vi "Calulate Fluid Level.vi"(8 "error in (no error)":errorcluster, 11 "Model Data":T1) -> (0 "error out":errorcluster, 3 "Model Data Out":T1)   [LabVIEW 2016, in "Model.lvlib"]
uses:
  Model.lvlib
  TypeDefs/Model Data.ctl
  TypeDefs/PL Settings.ctl
  TypeDefs/PL UI Refs.ctl
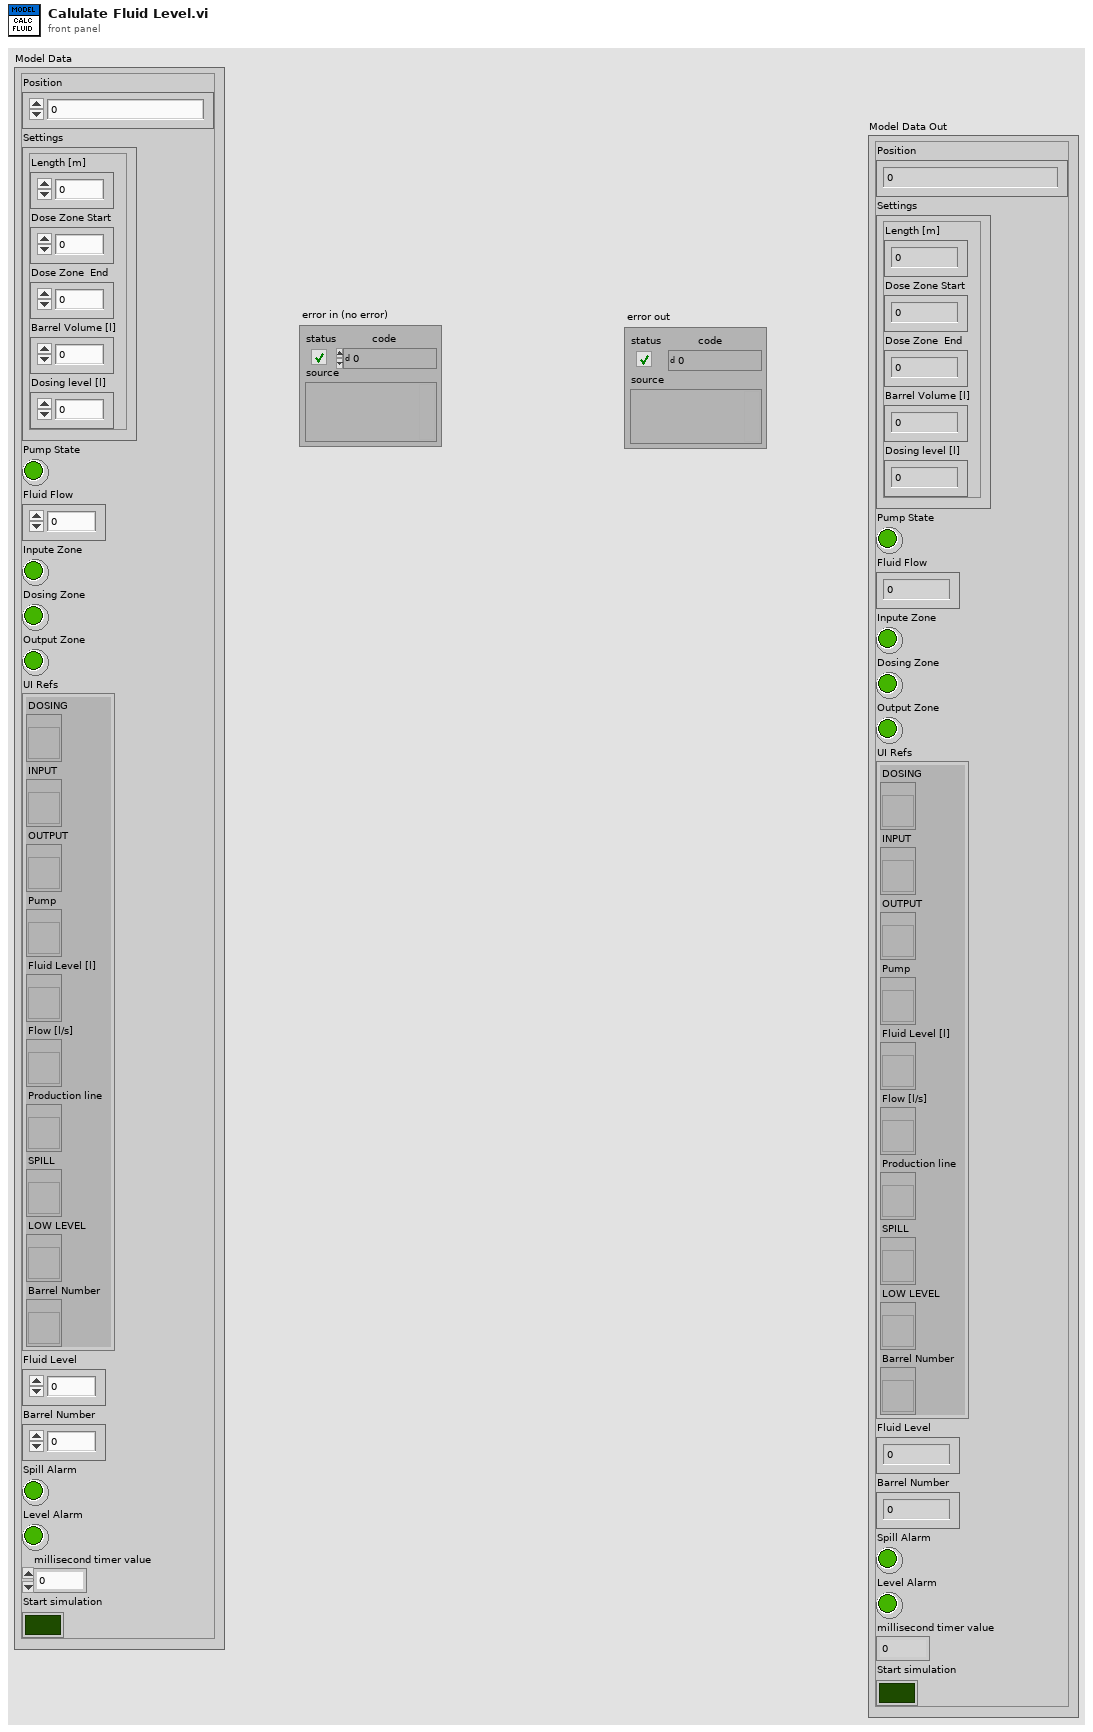
[diagram p1: front panel]
types:
  T1 = typedef "Model.lvlib/Model Data.ctl" = cluster{"Position":dbl, "Settings":T2, "Pump State":bool, "Fluid Flow":dbl, "Inpute Zone":bool, "Dosing Zone":bool, "Output Zone":bool, "UI Refs":T3, "Fluid Level":dbl, "Barrel Number":i32, "Spill Alarm":bool, "Level Alarm":bool, "millisecond timer value":u32, "Start simulation":bool}
  T2 = typedef "Model.lvlib/PL Settings.ctl" = cluster{"Length [m]":dbl, "Dose Zone Start":dbl, "Dose Zone  End":dbl, "Barrel Volume [l]":dbl, "Dosing level [l]":dbl}
  T3 = typedef "Model.lvlib/PL UI Refs.ctl" = cluster{"DOSING":refnum<vi>, "INPUT":refnum<vi>, "OUTPUT":refnum<vi>, "Pump":refnum<vi>, "Fluid Level [l]":refnum<vi>, "Flow [l/s]":refnum<vi>, "Production line":refnum<vi>, "SPILL":refnum<vi>, "LOW LEVEL":refnum<vi>, "Barrel Number":refnum<vi>}
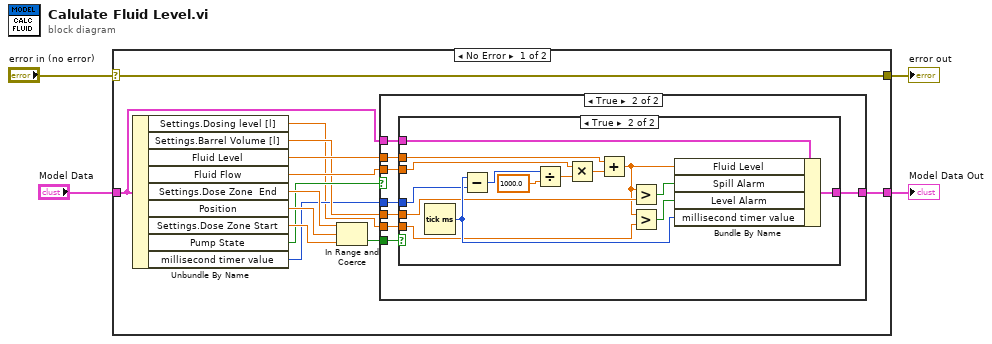
[diagram p0: block diagram]
diagram:
  n1 = case shown="No Error" "error in (no error)" {
    selector: "error in (no error)" -> [w8 w44]
    tunnel: "Model Data" -> [w10 w43]
    tunnel: [w9 w43] -> w3
    tunnel: [w8 w44] -> w1
    frame No Error {
      n2 = Unbundle By Name(w10) -> ("Settings.Dosing level [l]"=w5:dbl, "Settings.Barrel Volume [l]"=w7:dbl, "Fluid Level"=w11:dbl, "Fluid Flow"=w12:dbl, "Settings.Dose Zone  End"=w17:dbl, "Position"=w16:dbl, "Settings.Dose Zone Start"=w15:dbl, "Pump State"=w14:bool, "millisecond timer value"=w6:u32)
      n3 = In Range and Coerce(upper limit=w17, x=w16, lower limit=w15) -> (In Range?=w13:bool)  [unwired: 1 out]
      n4 = case shown="True" w14 {
        tunnel: w13 -> [_ w26]
        tunnel: w12 -> [_ w25]
        tunnel: w11 -> [_ w24]
        tunnel: w10 -> [w18 w23]
        tunnel: [w18 w22] -> w9
        tunnel: w7 -> [_ w21]
        tunnel: w6 -> [_ w20]
        tunnel: w5 -> [_ w19]
        frame False {
        }
        frame True {
          n5 = case shown="True" w26 {
            tunnel: w25 -> [_ w34]
            tunnel: w24 -> [_ w29]
            tunnel: w23 -> [w27 w42]
            tunnel: [w27 w41] -> w22
            tunnel: w21 -> [_ w32]
            tunnel: w20 -> [_ w38]
            tunnel: w19 -> [_ w31]
            frame False {
            }
            frame True {
              n6 = Tick Count (ms)() -> (millisecond timer value=w39:u32)
              n7 = Subtract(x=w39, y=w38) -> (x-y=w37:u32)
              n8 = Divide(x=w37, y=1000.0) -> (x/y=w36:dbl)
              n9 = Multiply(x=w34, y=w36) -> (x*y=w33:dbl)
              n10 = Add(x=w29, y=w33) -> (x+y=w28:dbl)
              n11 = Greater?(x=w28, y=w32) -> (0:w40:bool)
              n12 = Greater?(x=w28, y=w31) -> (0:w30:bool)
              n13 = Bundle By Name(cluster=w42, "Fluid Level"=w28, "Spill Alarm"=w40, "Level Alarm"=w30, "millisecond timer value"=w39) -> (w41:T1)
            }
          }
        }
      }
    }
    frame Error {
    }
  }
  "Model Data Out" <- w3
  "error out" <- w1
